vi "Stop BuildWorker.vi"(8 "error in (no error)":errorcluster, 11 "BuildWorker Controller in":refnum<class "BuildWorker Controller.lvclass">) -> (0 "error out":errorcluster, 3 "BuildWorker Controller out":refnum<class "BuildWorker Controller.lvclass">)   [LabVIEW 2017, in "BuildWorker Controller.lvclass"]
uses:
  BuildWorker Controller.lvclass
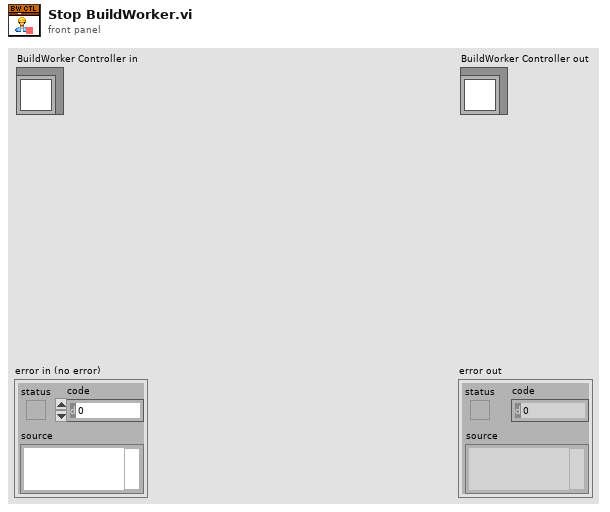
[diagram p1: front panel]
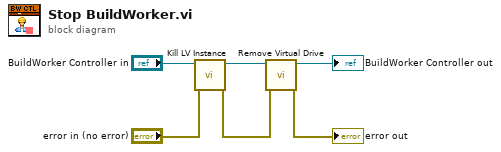
[diagram p0: block diagram]
diagram:
  n1 = call "Kill LV Instance.vi"("error in (no error)"="error in (no error)", "BuildWorker Controller in"="BuildWorker Controller in") -> ("error out"=w2:errorcluster, "BuildWorker Controller out"=w5:refnum<class "BuildWorker Controller.lvclass">)  [unwired: 8 in]
  n2 = call "Remove Virtual Drive.vi"("error in (no error)"=w2, "BuildWorker Controller in"=w5) -> ("error out"=→"error out":errorcluster, "BuildWorker Controller out"=→"BuildWorker Controller out":refnum<class "BuildWorker Controller.lvclass">)  [unwired: 8 in]
